vi "Create Array from FQN.vi"(1 "FQN In":string="Fcn_AcqVoltage.lvlib:Fcn_AcqVoltage.lvclass:Read RESOLUTION_TYPE.vi") -> (0 "Array of namespaces and name":string[](array[string]))   [LabVIEW 2018, in "Path and String Processing.lvlib"]
uses:
  Path and String Processing.lvlib
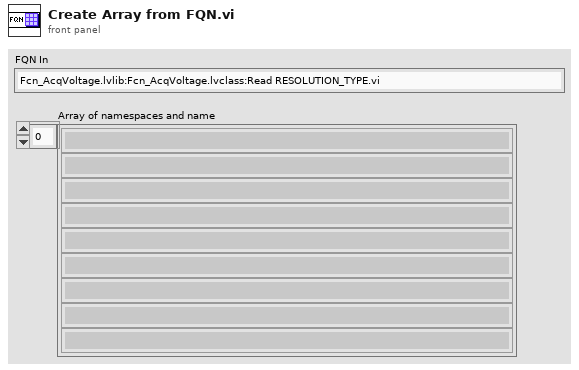
[diagram p1: front panel]
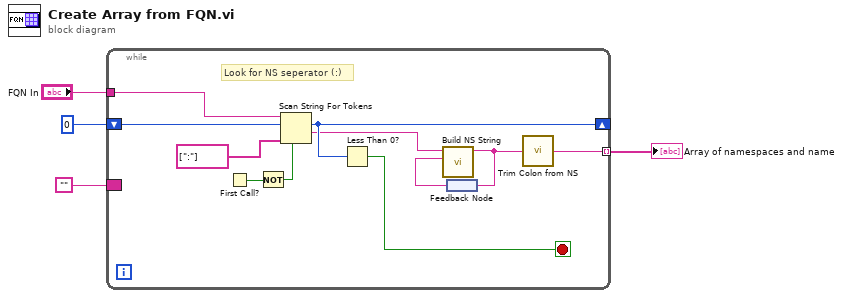
[diagram p0: block diagram]
diagram:
  n1 = while {
    tunnel: "FQN In" -> [w15]
    shift-right: [w11] -> _
    shift-left: 0 ("offset past token") -> [w13]
    tunnel: [w12] -> w2 mode=indexing
    border: "" ("Current Namespace loopback") -> [_]
    stop <- w14 stop-if-true
    # "Look for NS seperator (:)"
    n2 = First Call?() -> (First Call?: T/F=w5:bool)
    n3 = Not(x=w5) -> (.not. x?=w7:bool)
    n4 = Scan String For Tokens(4:w7, 6:string[] [":"] ("delimiters (\\s,\\t,\\r,\\n)"), 8:w13, 9:w15) -> (1:w10:string, 2:w11:i32)  [unwired: 2 in, 2 out]
    n5 = Less Than 0?(x=w11) -> (x < 0?=w14:bool)
    n6 = feedback #1() -> (w9:string)
    n7 = call "Build NS String.vi"("Previous Namespaces"=w9, "Namespace name"=w10) -> ("New Namespace string"=w8:string)  [unwired: 9 in]
    n8 = feedback-in #1(w8) -> ()
    n9 = call "Trim Colon from NS.vi"("String in"=w8) -> ("String out"=w12:string)
  }
  "Array of namespaces and name" <- w2
